vi "Hysterisis.vi"(0 "Low to High\nTransition":sgl(knob)=0.70161825 scale=0.0..1.0, 1 "Sample Size":i32=5, 2 "New Sample":sgl, 3 "High to Low\nTransition":sgl(knob)=0.29833332 scale=0.0..1.0, 4 "Initial State":bool) -> (7 "Output":bool)   [LabVIEW 2013]
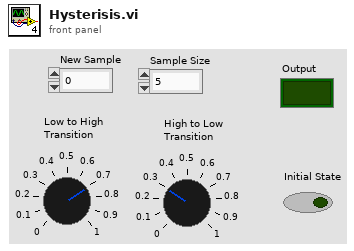
[diagram p1: front panel]
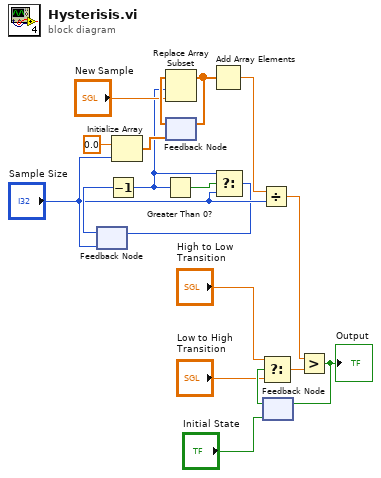
[diagram p0: block diagram]
diagram:
  n1 = feedback #1("Sample Size") -> (w12:i32)
  n2 = Decrement(x=w12) -> (x-1=w8:i32)
  n3 = Initialize Array(sgl 0.0, "Sample Size") -> (w17:sgl[])
  n4 = Greater Than 0?(x=w8) -> (x > 0?=w11:bool)
  n5 = feedback #2(w17) -> (w14:sgl[])
  n6 = Replace Array Subset(array=w14, new element="New Sample", index=w8) -> (w1:sgl[])
  n7 = feedback-in #2(w1) -> ()
  n8 = Add Array Elements(numeric array=w1) -> (sum=w18:sgl)
  n9 = Select(t=w8, s=w11, f="Sample Size") -> (s? t:f=w9:i32)
  n10 = feedback-in #1(w9) -> ()
  n11 = Divide(x=w18, y="Sample Size") -> (x/y=w7:sgl)
  n12 = feedback #3("Initial State") -> (w5:bool)
  n13 = Select(t="High to Low\nTransition", s=w5, f="Low to High\nTransition") -> (s? t:f=w6:sgl)
  n14 = Greater?(x=w7, y=w6) -> (0:w2:bool)
  "Output" <- w2
  n15 = feedback-in #3(w2) -> ()
